vi "FTW-JSON-Container-JsonType.vi"(7 "Container":refnum<class "FTW-Container.lvclass">) -> (8 "JSON Element Type":T1)   [LabVIEW 2015]
uses:
  FTW-JSON-Type.ctl
  container/FTW-Container.lvclass
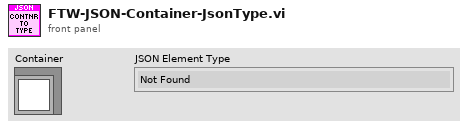
[diagram p1: front panel]
types:
  T1 = typedef "FTW-JSON-Type.ctl" = enum8{"Not Found", "Object", "Array", "String", "Number", "Boolean", "null"}
  T2 = typedef "NI_Data Type.lvlib/Data Type.ctl" = enum8{"Invalid Type", "Void", "I8", "I16", "I32", "I64", "U8", "U16", "U32", "U64", "Single Float", "Double Float", "Extended Float", "Single Complex", "Double Complex", "Extended Complex", "Enum U8", "Enum U16", "Enum U32", "Enum U64", "Single Float With Unit", "Double Float With Unit", "Extended Float With Unit", "Single Complex with Unit", "Double Complex with Unit", "Extended Complex with Unit", "Boolean", "String", "Path", "Picture", "Tag", "Array", "Cluster", "Variant", "LV Variant", "Waveform", "Timestamp", "Digital Waveform", "Digital Data", "ExpressData", "Refnum", "External Data", "VI", "Poly VI", "LabVIEW Class Instance", "Fixed Point"}
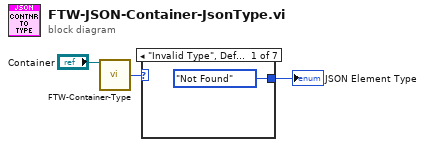
[diagram p0: block diagram]
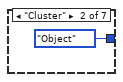
[diagram p2: hidden frame]
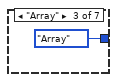
[diagram p3: hidden frame]
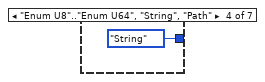
[diagram p4: hidden frame]
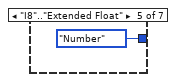
[diagram p5: hidden frame]
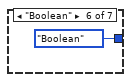
[diagram p6: hidden frame]
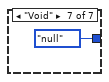
[diagram p7: hidden frame]
diagram:
  n1 = call "FTW-Container-Type.vi"("FTW-Container In"="Container") -> ("Type"=w2:T2)  [unwired: 12 in, 2 out]
  n2 = case shown="\"Invalid Type\", Default" w2 {
    tunnel: [FTW-JSON-Type."Not Found" ("JSON Element Type") FTW-JSON-Type."Object" ("JSON Element Type") FTW-JSON-Type."Array" ("JSON Element Type") FTW-JSON-Type."String" ("JSON Element Type") FTW-JSON-Type."Number" ("JSON Element Type") FTW-JSON-Type."Boolean" ("JSON Element Type") FTW-JSON-Type."null" ("JSON Element Type")] -> w3
    frame "Invalid Type", Default {
    }
    frame "Cluster" {
    }
    frame "Array" {
    }
    frame "Enum U8".."Enum U64", "String", "Path" {
    }
    frame "I8".."Extended Float" {
    }
    frame "Boolean" {
    }
    frame "Void" {
    }
  }
  "JSON Element Type" <- w3
